vi "parallel_reg.vi"(0 "RD":bool, 1 "I":T3, 2 "C":bool, 3 "R":bool, 4 "WR":bool) -> (5 "O":T1, 6 "direct_out":T1)   [LabVIEW 2013]
panel:
  in  "S":T2
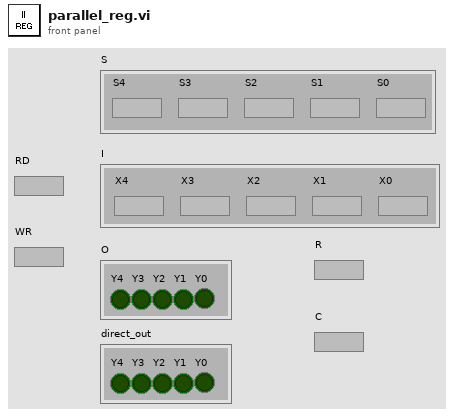
[diagram p1: front panel]
types:
  T1 = cluster{"Y4":bool, "Y3":bool, "Y2":bool, "Y1":bool, "Y0":bool}
  T2 = cluster{"S4":bool, "S3":bool, "S2":bool, "S1":bool, "S0":bool}
  T3 = cluster{"X4":bool, "X3":bool, "X2":bool, "X1":bool, "X0":bool}
  T4 = cluster{"Q":bool, "Q":bool, "Q":bool, "Q":bool, "Q":bool}
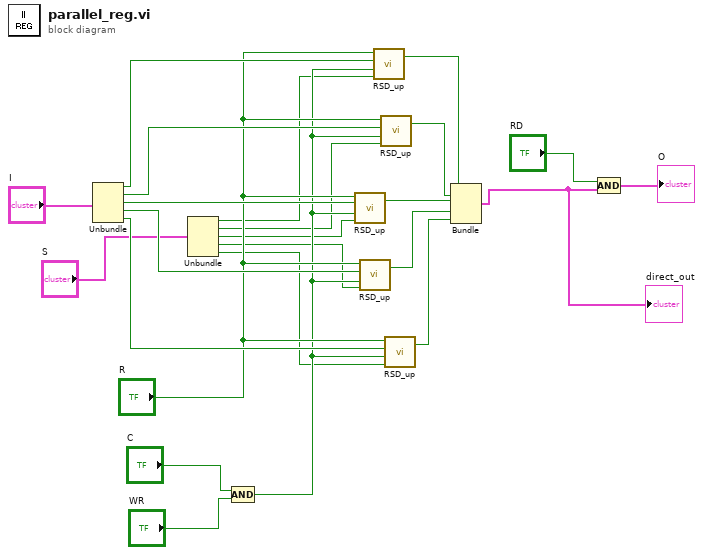
[diagram p0: block diagram]
diagram:
  n1 = Unbundle("I") -> ("X4"=w24:bool, "X3"=w23:bool, "X2"=w22:bool, "X1"=w21:bool, "X0"=w20:bool)
  n2 = Unbundle("S") -> ("S4"=w6:bool, "S3"=w5:bool, "S2"=w4:bool, "S1"=w3:bool, "S0"=w2:bool)
  n3 = Compound Arithmetic op=AND("C", "WR") -> (w10:bool)
  n4 = call "RSD_up.vi"("S"=w4, "C"=w10, "D"=w22, "R"="R") -> ("Q"=w13:bool)  [unwired: 1 out]
  n5 = call "RSD_up.vi"("S"=w3, "C"=w10, "D"=w21, "R"="R") -> ("Q"=w17:bool)  [unwired: 1 out]
  n6 = call "RSD_up.vi"("S"=w6, "C"=w10, "D"=w24, "R"="R") -> ("Q"=w18:bool)  [unwired: 1 out]
  n7 = call "RSD_up.vi"("S"=w5, "C"=w10, "D"=w23, "R"="R") -> ("Q"=w19:bool)  [unwired: 1 out]
  n8 = call "RSD_up.vi"("S"=w2, "C"=w10, "D"=w20, "R"="R") -> ("Q"=w16:bool)  [unwired: 1 out]
  n9 = Bundle("Q"=w18, "Q"=w19, "Q"=w13, "Q"=w17, "Q"=w16) -> (w1:T4)  [unwired: 1 in]
  "direct_out" <- w1
  n10 = Compound Arithmetic op=AND("RD", w1) -> (→"O":T4)
